vi "ToRepo.vi"(8 "error in":errorcluster, 9 "to repo cluster":T1, 10 "repository in":refnum<class "NISE_CEF_Repository.lvclass">, 11 "group in":refnum<class "Group.lvclass">) -> (0 "error out":errorcluster, 2 "repository out":refnum<class "NISE_CEF_Repository.lvclass">, 3 "group out":refnum<class "Group.lvclass">)   [LabVIEW 2015, in "Group.lvclass"]
uses:
  Group.lvclass
  <vilib>/NI/Configuration Framework/Repository/NISE_CEF_Repository.lvclass
  <vilib>/NI/Configuration Framework/Node/ToRepoCluster.ctl
  cRIO Repo/cRIORepo.lvclass
  Group.lvclass/Group.ctl
  cRIO Repo/cRIORepo.lvclass/cRIORepo.ctl
  Read GroupName.vi
  cRIO Repo/Write Channel Group.vi
  <vilib>/NI/Configuration Framework/Node/NISE_CEF_Node.lvclass
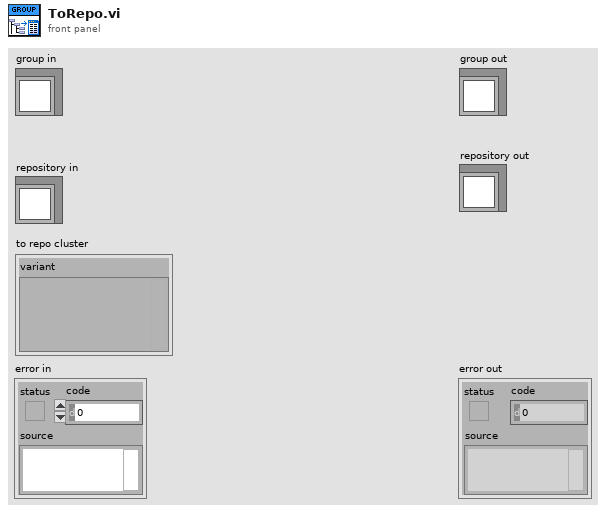
[diagram p1: front panel]
types:
  T1 = typedef "NISE_CEF_Node.lvclass/ToRepoCluster.ctl" = cluster{"variant":variant}
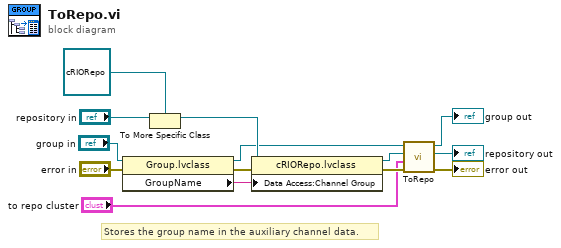
[diagram p0: block diagram]
diagram:
  # "Stores the group name in the auxiliary channel data."
  n1 = property class="Group.lvclass"(reference="group in", error in="error in") -> (reference out=w7:refnum<class "Group.lvclass">, error out=w3:errorcluster, "GroupName"=w9:string)
  n2 = To More Specific Class(target class=refnum<class "cRIORepo.lvclass"> refnum ("cRIO repo.lvclass"), reference="repository in") -> (specific class reference=w10:refnum<class "cRIORepo.lvclass">)  [unwired: 1 in, 1 out]
  n3 = property class="cRIORepo.lvclass"(reference=w10, error in=w3, "Data Access:Channel Group"=w9) -> (reference out=w5:refnum<class "cRIORepo.lvclass">, error out=w2:errorcluster)
  n4 = call-parent "ToRepo.vi"("error in"=w2, "to repo cluster"="to repo cluster", "repository in"=w5, "node in"=w7) -> ("error out"=→"error out":errorcluster, "repository out"=→"repository out":refnum<class "NISE_CEF_Repository.lvclass">, "node out"=→"group out":refnum<class "Group.lvclass">)  [unwired: 5 in]
